vi "Write PowerData.vi"(8 "error in (no error)":errorcluster, 10 "PowerData":T1, 11 "SetPower Message":refnum<class "SetPower Message.lvclass">) -> (0 "error out":errorcluster, 3 "SetPower Message":refnum<class "SetPower Message.lvclass">)   [LabVIEW 2018, in "QMH_Class.lvlib" / "TestManager.lvlib" / "SetPower Message.lvclass"]
uses:
  SetPower Message.lvclass
  SetPower Message.lvclass/SetPower Message.ctl
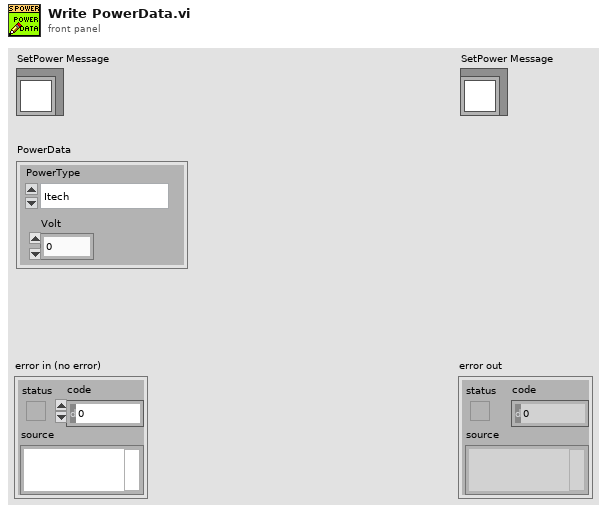
[diagram p1: front panel]
types:
  T1 = cluster{"Volt":dbl, "PowerType":enum16{"Itech", "Keysight"}}
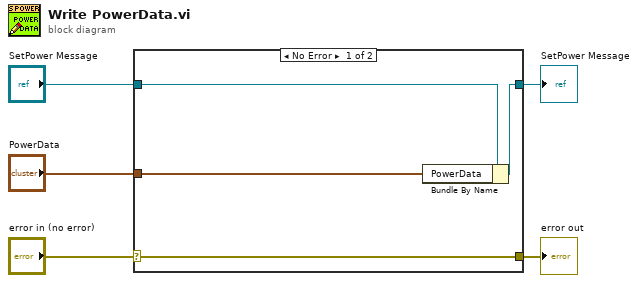
[diagram p0: block diagram]
diagram:
  n1 = case shown="No Error" "error in (no error)" {
    selector: "error in (no error)" -> [w9 w10]
    tunnel: [w9 w10] -> w4
    tunnel: [w7 w11] -> w2
    tunnel: "SetPower Message" -> [w8 w11]
    tunnel: "PowerData" -> [w6 _]
    frame No Error {
      n2 = Bundle By Name(cluster=w8, "PowerData"=w6) -> (w7:refnum<class "SetPower Message.lvclass">)
    }
    frame Error {
    }
  }
  "error out" <- w4
  "SetPower Message" <- w2
